vi "InterfaceAODSWWithStabilizationSW.vi"(6 "Y-Z Motion Points":i32[][](array[numeric]), 7 "X-Y Motion Points":i32[][](array[numeric]), 8 "Grid Points":dbl, 9 "Motion Points":dbl, 10 "Scan Info":T1, 11 "Data":i32[][](array[numeric])) -> (2 "Number of Planes":dbl, 3 "Array":cluster{dbl[][], dbl, dbl, dbl, dbl, dbl, dbl}[](array[cluster]))   [LabVIEW 2014]
uses:
  <vilib>/Analysis/NI_AALBase.lvlib
panel:
  out "dz_YZ":dbl
  out "dy_XY":dbl
  out "dx_XY":dbl
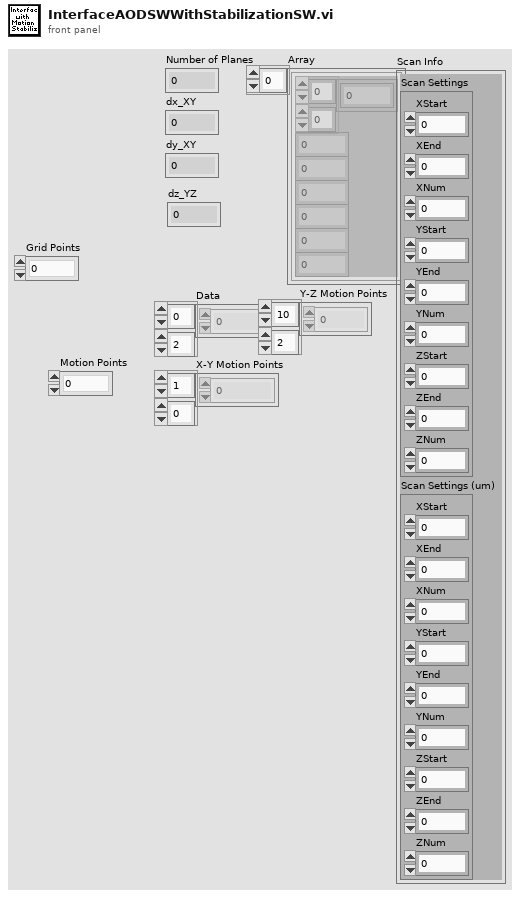
[diagram p1: front panel]
types:
  T1 = cluster{"Scan Settings":cluster{"XStart":i32, "XEnd":i32, "XNum":i32, "YStart":i32, "YEnd":i32, "YNum":i32, "ZStart":i32, "ZEnd":i32, "ZNum":i32}, "Scan Settings (um)":cluster{"XStart":i32, "XEnd":i32, "XNum":i32, "YStart":i32, "YEnd":i32, "YNum":i32, "ZStart":i32, "ZEnd":i32, "ZNum":i32}}
  T2 = cluster{"XStart":i32, "XEnd":i32, "XNum":i32, "YStart":i32, "YEnd":i32, "YNum":i32, "ZStart":i32, "ZEnd":i32, "ZNum":i32}
  T3 = cluster{dbl[][], dbl, dbl, dbl, dbl, dbl, "dz_YZ":dbl}
  T4 = cluster{dbl[][], dbl, "dy_XY":dbl, dbl, "dx_XY":dbl, dbl, dbl}
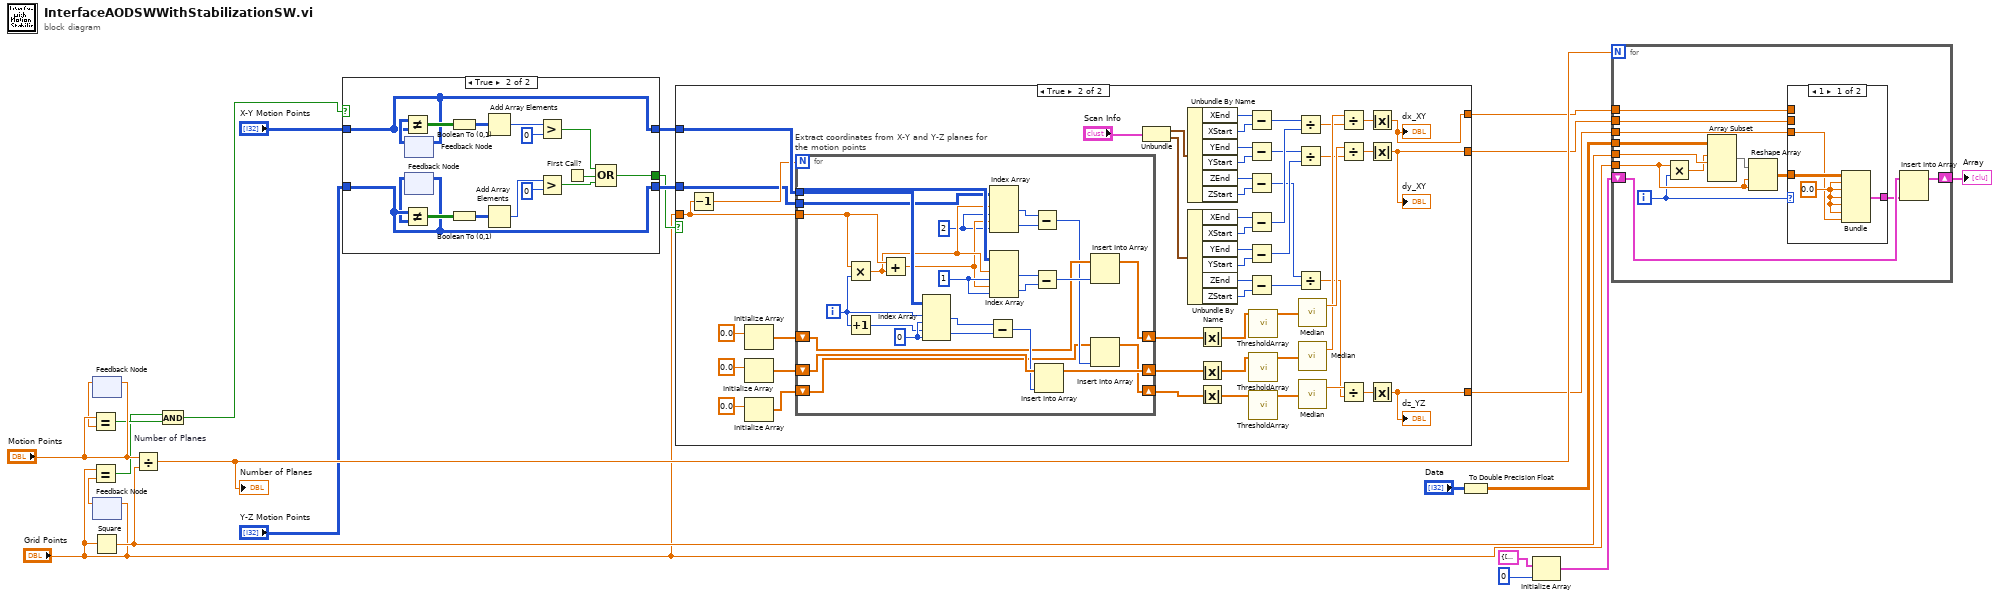
[diagram p0: block diagram]
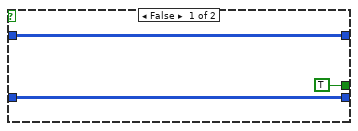
[diagram p2: hidden frame]
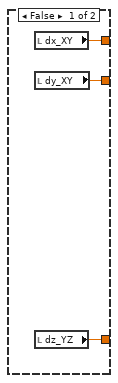
[diagram p3: hidden frame]
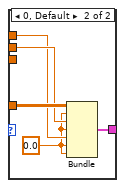
[diagram p4: hidden frame]
diagram:
  n1 = Square(x="Grid Points") -> (x^2=w17:dbl)
  n2 = feedback-in #1("Motion Points") -> ()
  n3 = feedback #1() -> (w7:dbl)  [unwired: 1 in]
  n4 = Equal?(x="Motion Points", y=w7) -> (x = y?=w5:bool)
  n5 = feedback-in #2("Grid Points") -> ()
  n6 = feedback #2() -> (w9:dbl)  [unwired: 1 in]
  n7 = Equal?(x="Grid Points", y=w9) -> (x = y?=w4:bool)
  n8 = Divide "Number of Planes"(x="Motion Points", y=w17) -> (x/y=w23:dbl)
  "Number of Planes" <- w23
  n9 = And(x=w4, y=w5) -> (x .and. y?=w6:bool)
  n10 = case shown="True" w6 {
    tunnel: [w26 w27] -> w12
    tunnel: [w25 w30] -> w11
    tunnel: [TRUE w31] -> w10
    tunnel: "X-Y Motion Points" -> [w26 w27]
    tunnel: "Y-Z Motion Points" -> [w25 w30]
    frame False {
    }
    frame True {
      n11 = feedback #3() -> (w28:i32[][])  [unwired: 1 in]
      n12 = Not Equal?(x=w28, y=w27) -> (x != y?=w42:bool[][])
      n13 = feedback-in #3(w27) -> ()
      n14 = feedback #4() -> (w29:i32[][])  [unwired: 1 in]
      n15 = Not Equal?(x=w30, y=w29) -> (x != y?=w38:bool[][])
      n16 = feedback-in #4(w30) -> ()
      n17 = Boolean To (0,1)(Boolean=w42) -> (0, 1=w41:i16[][])
      n18 = Boolean To (0,1)(Boolean=w38) -> (0, 1=w37:i16[][])
      n19 = Add Array Elements(numeric array=w41) -> (sum=w40:i16)
      n20 = Add Array Elements(numeric array=w37) -> (sum=w36:i16)
      n21 = Greater?(x=w40, y=i16 0) -> (0:w33:bool)
      n22 = Greater?(x=w36, y=i16 0) -> (0:w32:bool)
      n23 = First Call?() -> (First Call?: T/F=w34:bool)
      n24 = Compound Arithmetic op=OR(w33, w34, w32) -> (w31:bool)
    }
  }
  n25 = case shown="True" w10 {
    tunnel: w12 -> [_ w58]
    tunnel: w11 -> [_ w49]
    tunnel: [w44 w59] -> w15
    tunnel: [w43 w60] -> w13
    tunnel: [w45 w61] -> w14
    tunnel: "Grid Points" -> [_ w51]
    frame False {
      n26 = local read "dx_XY"() -> (w45:dbl)
      n27 = local read "dy_XY"() -> (w43:dbl)
      n28 = local read "dz_YZ"() -> (w44:dbl)
    }
    frame True {
      n29 = Decrement(x=w51) -> (x-1=w54:dbl)
      n30 = Initialize Array(0.0 ("element")) -> (w52:dbl[])  [unwired: 1 in]
      n31 = Initialize Array(0.0 ("element")) -> (w56:dbl[])  [unwired: 1 in]
      n32 = Initialize Array(0.0 ("element")) -> (w47:dbl[])  [unwired: 1 in]
      n33 = for "Extract coordinates from X-Y and Y-Z planes for the motion points" {
        N: w54 -> [_]
        tunnel: w58 -> [w110]
        shift-right: [w117] -> w55
        shift-left: w56 -> [w118]
        shift-right: [w111] -> w50
        shift-left: w52 -> [w112]
        tunnel: w51 -> [w108]
        tunnel: w49 -> [w103]
        shift-right: [w98] -> w46
        shift-left: w47 -> [w99]
        i -> [w109]
        w104 = 2 ("index (col)")
        w107 = 1 ("disabled index (col)")
        w122 = 0 ("disabled index (col)")
        n34 = Multiply(x=w108, y=w109) -> (x*y=w106:dbl)
        n35 = Increment(x=w109) -> (x+1=w121:i32)
        n36 = Add(x=w108, y=w106) -> (x+y=w105:dbl)
        n37 = Index Array(array=w110, index (row) #1=w109, index (col) #1=w122, index (row) #2=w121, index (col) #2=w122) -> (element #1=w120:i32, element #2=w119:i32)
        n38 = Subtract(x=w120, y=w119) -> (x-y=w116:i32)
        n39 = Index Array(array=w103, index (row) #1=w106, index (col) #1=w104, index (row) #2=w105, index (col) #2=w104) -> (element #1=w102:i32, element #2=w101:i32)
        n40 = Index Array(array=w110, index (row) #1=w106, index (col) #1=w107, index (row) #2=w105, index (col) #2=w107) -> (element #1=w115:i32, element #2=w114:i32)
        n41 = Subtract(x=w102, y=w101) -> (x-y=w100:i32)
        n42 = Subtract(x=w115, y=w114) -> (x-y=w113:i32)
        n43 = Insert Into Array(array=w118, new element=w116) -> (w117:dbl[])  [unwired: 1 in]
        n44 = Insert Into Array(array=w112, new element=w113) -> (w111:dbl[])  [unwired: 1 in]
        n45 = Insert Into Array(array=w99, new element=w100) -> (w98:dbl[])  [unwired: 1 in]
      }
      n46 = Unbundle("Scan Info") -> ("Scan Settings"=w96:T2, "Scan Settings (um)"=w89:T2)
      n47 = Unbundle By Name(w96) -> ("XEnd"=w95:i32, "XStart"=w94:i32, "YEnd"=w93:i32, "YStart"=w92:i32, "ZEnd"=w91:i32, "ZStart"=w90:i32)
      n48 = Unbundle By Name(w89) -> ("XEnd"=w88:i32, "XStart"=w87:i32, "YEnd"=w86:i32, "YStart"=w85:i32, "ZEnd"=w84:i32, "ZStart"=w83:i32)
      n49 = Absolute Value(x=w50) -> (abs(x)=w63:dbl[])
      n50 = Absolute Value(x=w55) -> (abs(x)=w64:dbl[])
      n51 = Absolute Value(x=w46) -> (abs(x)=w62:dbl[])
      n52 = Subtract(x=w95, y=w94) -> (x-y=w82:i32)
      n53 = Subtract(x=w93, y=w92) -> (x-y=w80:i32)
      n54 = Subtract(x=w91, y=w90) -> (x-y=w78:i32)
      n55 = Subtract(x=w88, y=w87) -> (x-y=w81:i32)
      n56 = Subtract(x=w86, y=w85) -> (x-y=w79:i32)
      n57 = Subtract(x=w84, y=w83) -> (x-y=w77:i32)
      n58 = call "ThresholdArray.vi"("Input Array"=w63) -> ("Thresholded Array"=w67:dbl[])  [unwired: 10 in]
      n59 = call "ThresholdArray.vi"("Input Array"=w64) -> ("Thresholded Array"=w68:dbl[])  [unwired: 10 in]
      n60 = call "ThresholdArray.vi"("Input Array"=w62) -> ("Thresholded Array"=w66:dbl[])  [unwired: 10 in]
      n61 = Divide(x=w82, y=w81) -> (x/y=w71:dbl)
      n62 = Divide(x=w80, y=w79) -> (x/y=w70:dbl)
      n63 = Divide(x=w78, y=w77) -> (x/y=w69:dbl)
      n64 = call <vilib>:"Median.vi"("X"=w67) -> ("median"=w74:dbl)  [unwired: 1 out]
      n65 = call <vilib>:"Median.vi"("X"=w68) -> ("median"=w73:dbl)  [unwired: 1 out]
      n66 = call <vilib>:"Median.vi"("X"=w66) -> ("median"=w72:dbl)  [unwired: 1 out]
      n67 = Divide(x=w73, y=w71) -> (x/y=w65:dbl)
      n68 = Divide(x=w74, y=w70) -> (x/y=w75:dbl)
      n69 = Divide(x=w72, y=w69) -> (x/y=w76:dbl)
      n70 = Absolute Value(x=w65) -> (abs(x)=w61:dbl)
      "dx_XY" <- w61
      n71 = Absolute Value(x=w75) -> (abs(x)=w60:dbl)
      "dy_XY" <- w60
      n72 = Absolute Value(x=w76) -> (abs(x)=w59:dbl)
      "dz_YZ" <- w59
    }
  }
  n73 = To Double Precision Float(number="Data") -> (double precision float=w22:dbl[][])
  n74 = Initialize Array(cluster{dbl[][], dbl, dbl, dbl, dbl, dbl, dbl} {[], 0.0, 0.0, 0.0, 0.0, 0.0, 0.0} ("output cluster"), 0 ("dimension size")) -> (w21:cluster{dbl[][], dbl, dbl, dbl, dbl, dbl, dbl}[])
  n75 = for {
    N: w23 -> [_]
    tunnel: w22 -> [w135]
    tunnel: "Grid Points" -> [w133]
    tunnel: w17 -> [w134]
    shift-right: [w131] -> w18
    shift-left: w21 -> [w132]
    tunnel: w14 -> [w124]
    tunnel: w15 -> [w125]
    tunnel: w13 -> [w130]
    i -> [w123]
    n76 = Multiply(x=w133, y=w123) -> (x*y=w129:dbl)
    n77 = Array Subset(array=w135, index (row)=w129, length (row)=w134) -> (w128:dbl[][])  [unwired: 2 in]
    n78 = Reshape Array(w128, w133, w133) -> (w127:dbl[][])
    n79 = case shown="1" w123 {
      tunnel: w130 -> [_ w142]
      tunnel: w124 -> [_ w141]
      tunnel: w127 -> [w138 w143]
      tunnel: [w139 w144] -> w126
      tunnel: w125 -> [w136 _]
      frame 1 {
        w137 = 0.0
        n80 = Bundle(w138, w137, w137, w137, w137, w137, "dz_YZ"=w136) -> (w139:T3)  [unwired: 1 in]
      }
      frame 0, Default {
        w140 = 0.0
        n81 = Bundle(w143, w140, "dy_XY"=w142, w140, "dx_XY"=w141, w140, w140) -> (w144:T4)  [unwired: 1 in]
      }
    }
    n82 = Insert Into Array(array=w132, new element=w126) -> (w131:cluster{dbl[][], dbl, dbl, dbl, dbl, dbl, dbl}[])  [unwired: 1 in]
  }
  "Array" <- w18
